vi "Poll.GlobalStop.Initialize.vi"(8 "error in (no error)":errorcluster) -> (0 "error out":errorcluster {"code" min=0 max=0}, 3 "Stop Ref":refnum<data-value>)   [LabVIEW 2019, in "OPC UA Client Engine.lvlib"]
uses:
  OPC UA Client Engine.lvlib
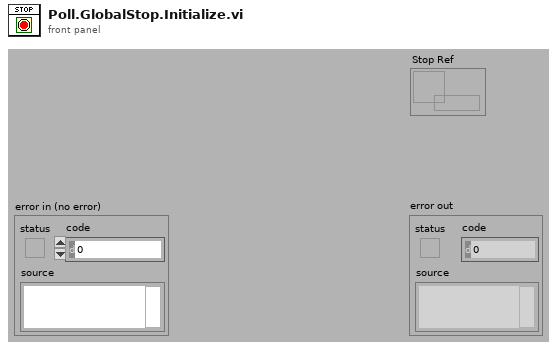
[diagram p1: front panel]
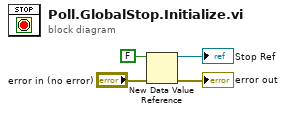
[diagram p0: block diagram]
diagram:
  n1 = New Data Value Reference(data value=FALSE, error in="error in (no error)") -> (data value reference=→"Stop Ref":refnum<data-value>, error out=→"error out":errorcluster)
